vi "acquire_data_errorHandler.vi"(8 "error in (no error)":errorcluster, 9 "length Sin wave Input":i32, 10 "input cluster":cluster{"z-err data":dbl[], "u_z-data":dbl[]}, 11 "Freq_i":dbl format="%#_13g") -> (0 "error out":errorcluster)   [LabVIEW 2017]
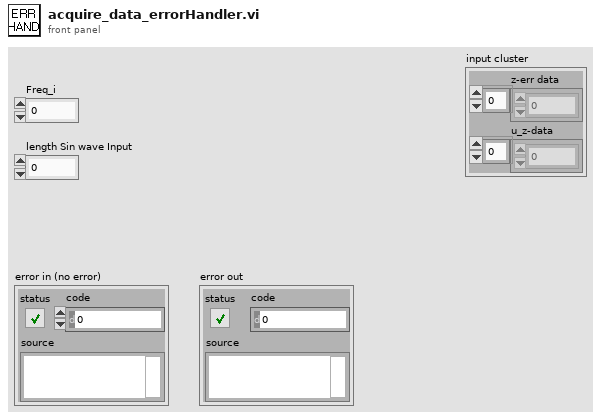
[diagram p1: front panel]
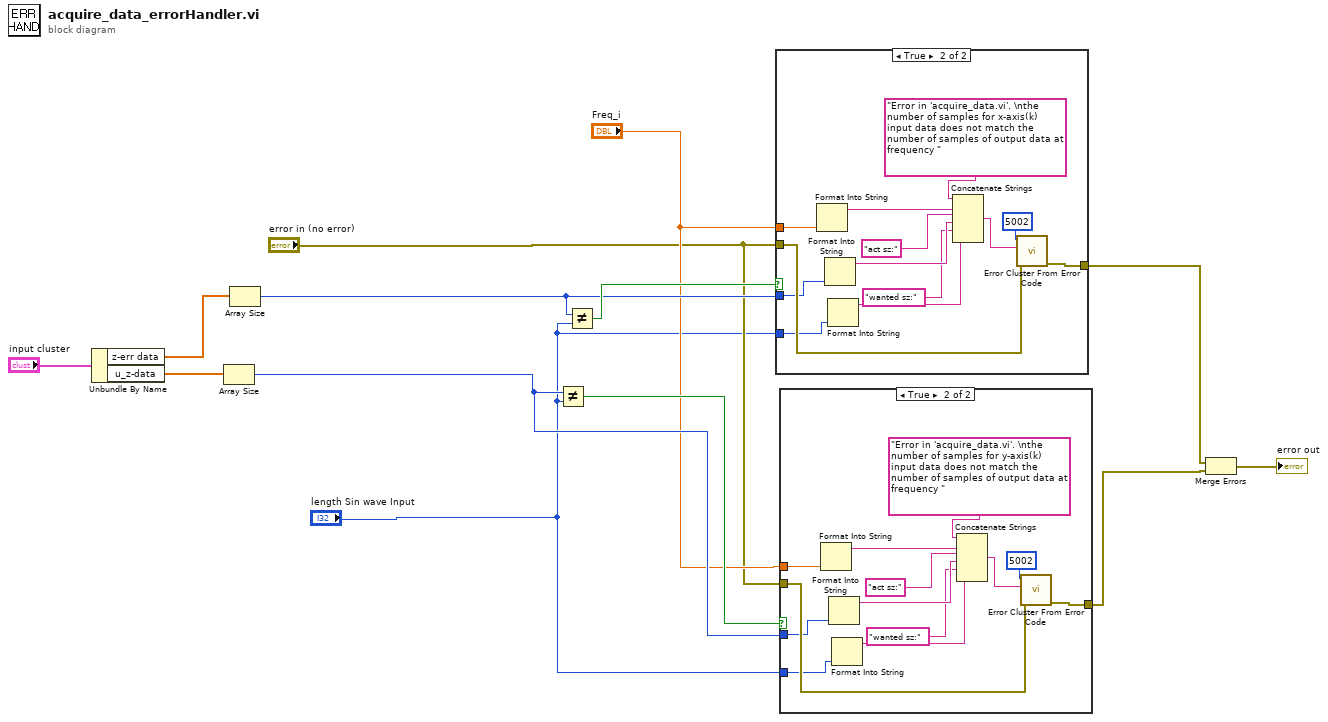
[diagram p0: block diagram]
diagram:
  n1 = Unbundle By Name("input cluster") -> ("z-err data"=w11:dbl[], "u_z-data"=w10:dbl[])
  n2 = Array Size(array=w10) -> (size(s)=w6:i32)
  n3 = Array Size(array=w11) -> (size(s)=w8:i32)
  n4 = Not Equal?(x=w6, y="length Sin wave Input") -> (x != y?=w7:bool)
  n5 = Not Equal?(x=w8, y="length Sin wave Input") -> (x != y?=w9:bool)
  n6 = case shown="True" w9 {
    tunnel: [w14 w27] -> w13
    tunnel: "error in (no error)" -> [w14 w22]
    tunnel: "Freq_i" -> [_ w21]
    tunnel: w8 -> [_ w16]
    tunnel: "length Sin wave Input" -> [_ w15]
    frame False {
    }
    frame True {
      n7 = Format Into String(w21) -> (resulting string=w25:string)  [unwired: 3 in, 1 out]
      n8 = Format Into String(w16) -> (resulting string=w19:string)  [unwired: 3 in, 1 out]
      n9 = Format Into String(w15) -> (resulting string=w17:string)  [unwired: 3 in, 1 out]
      n10 = Concatenate Strings("Error in 'acquire_data.vi'. \nthe number of samples for x-axis(k) input data does not match the number of samples of output data at frequency ", w25, "act sz:", w19, "wanted sz:", w17) -> (w24:string)
      n11 = call <vilib>:"Error Cluster From Error Code.vi"("error in (no error)"=w22, "error message (\"\")"=w24, "error code (0)"=5002) -> ("error out"=w27:errorcluster)  [unwired: 6 in]
    }
  }
  n12 = case shown="True" w7 {
    tunnel: [w28 w41] -> w2
    tunnel: "error in (no error)" -> [w28 w36]
    tunnel: "Freq_i" -> [_ w35]
    tunnel: w6 -> [_ w30]
    tunnel: "length Sin wave Input" -> [_ w29]
    frame False {
    }
    frame True {
      n13 = Format Into String(w35) -> (resulting string=w39:string)  [unwired: 3 in, 1 out]
      n14 = Format Into String(w30) -> (resulting string=w33:string)  [unwired: 3 in, 1 out]
      n15 = Format Into String(w29) -> (resulting string=w31:string)  [unwired: 3 in, 1 out]
      n16 = Concatenate Strings("Error in 'acquire_data.vi'. \nthe number of samples for y-axis(k) input data does not match the number of samples of output data at frequency ", w39, "act sz:", w33, "wanted sz:", w31) -> (w38:string)
      n17 = call <vilib>:"Error Cluster From Error Code.vi"("error in (no error)"=w36, "error message (\"\")"=w38, "error code (0)"=5002) -> ("error out"=w41:errorcluster)  [unwired: 6 in]
    }
  }
  n18 = Merge Errors(w13, w2) -> (→"error out":errorcluster)
